vi "BT Rx Test Get Default LSL.vi"(8 "error in (no error)":errorcluster, 11 "Template Tx Test in":refnum<class "niDTS BT Rx Test.lvclass">) -> (0 "error out":errorcluster, 2 "Default LSL":T1, 3 "Template Tx Test out":refnum<class "niDTS BT Rx Test.lvclass">)   [LabVIEW 2015, in "niDTS BT.lvlib" / "niDTS BT Rx Test.lvclass"]
uses:
  niDTS BT Rx Test.lvclass
  Includes/niDTS BT Rx Test INC Results.ctl
  niDTS BT Rx Test.lvclass/niDTS BT Rx Test.ctl
  Includes/niDTS BT INC Standard.ctl
  Includes/niDTS BT Rx Test INC Default Limits.vi
  niDTS BT.lvlib
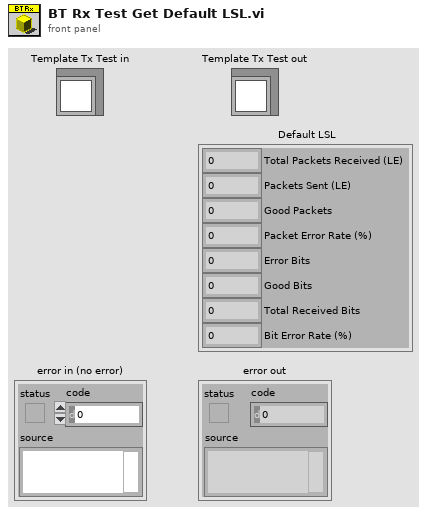
[diagram p1: front panel]
types:
  T1 = typedef "niDTS BT.lvlib/niDTS BT Rx Test INC Results.ctl" = cluster{"Total Packets Received (LE)":i32, "Packets Sent (LE)":dbl, "Good Packets":dbl, "Packet Error Rate (%)":dbl, "Error Bits":u32, "Good Bits":u32, "Total Received Bits":u32, "Bit Error Rate (%)":dbl}
  T2 = typedef "niDTS BT.lvlib/niDTS BT INC Standard.ctl" = enum16{"BDR", "EDR", "LE-TP"}
  T3 = typedef "niDTS BT.lvlib/niDTS BT INC Packet Type.ctl" = enum16{"NULL", "POLL", "FHS", "DM1", "DH1", "HV1", "HV2", "HV3", "EV3", "DV", "AUX1", "DM3", "DH3", "EV4", "EV5", "DM5", "DH5", "LE-TP"}
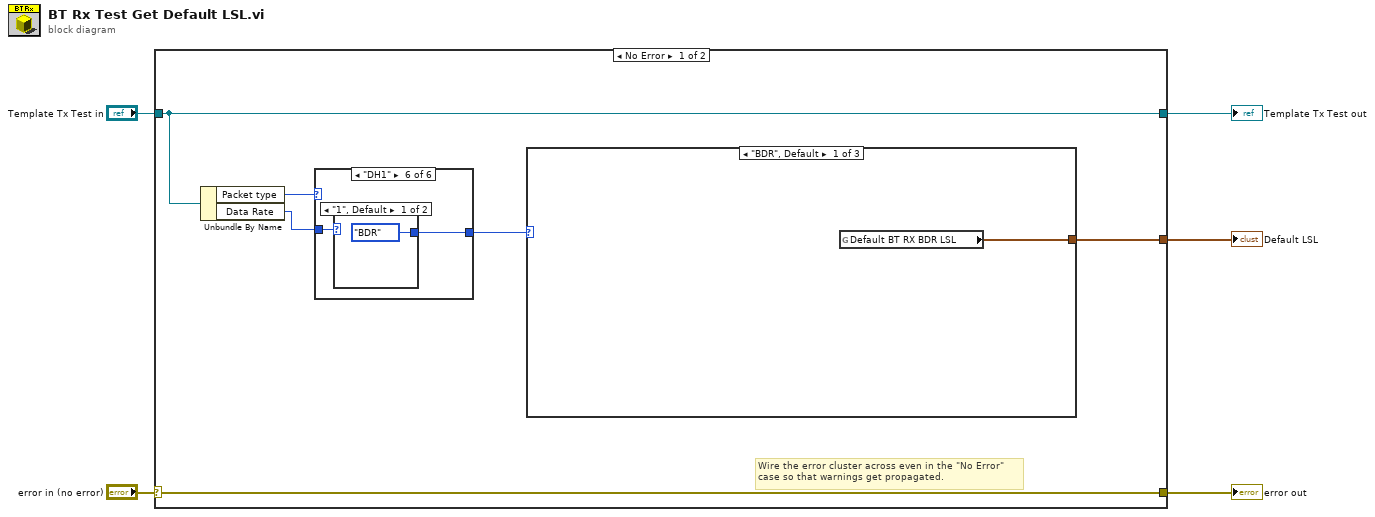
[diagram p0: block diagram]
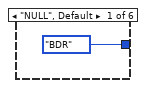
[diagram p2: hidden frame]
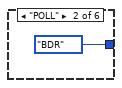
[diagram p3: hidden frame]
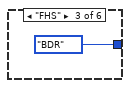
[diagram p4: hidden frame]
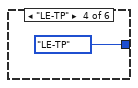
[diagram p5: hidden frame]
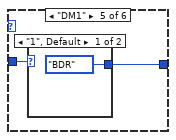
[diagram p6: hidden frame]
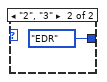
[diagram p7: hidden frame]
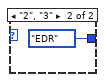
[diagram p8: hidden frame]
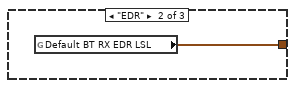
[diagram p9: hidden frame]
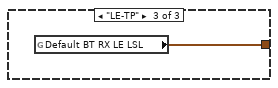
[diagram p10: hidden frame]
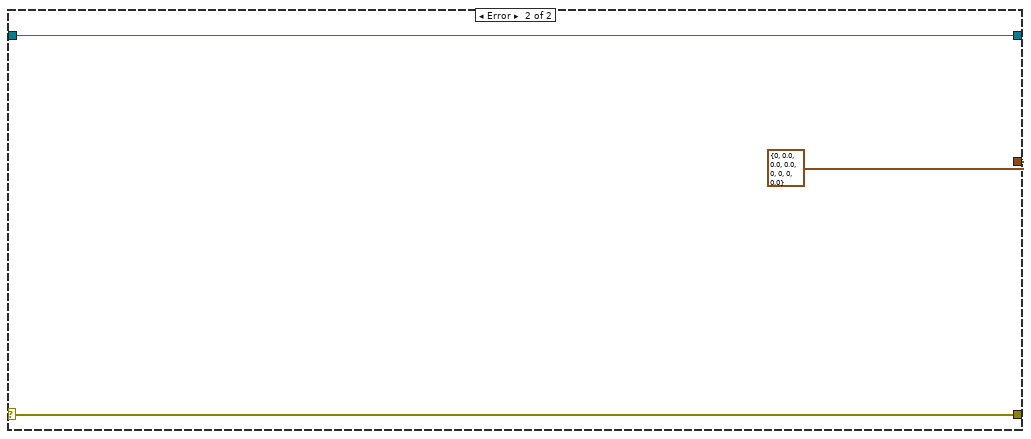
[diagram p11: hidden frame]
diagram:
  n1 = case shown="No Error" "error in (no error)" {
    selector: "error in (no error)" -> [w11 w29]
    tunnel: [w11 w29] -> w4
    tunnel: [w6 w28] -> w2
    tunnel: "Template Tx Test in" -> [w6 w28]
    tunnel: [w7 T1 {"Total Packets Received (LE)"=0, "Packets Sent (LE)"=0.0, "Good Packets"=0.0, "Packet Error Rate (%)"=0.0, "Error Bits"=0, "Good Bits"=0, "Total Received Bits"=0, "Bit Error Rate (%)"=0.0} ("Default LSL")] -> w1
    frame No Error {
      # "Wire the error cluster across even in the \"No Error\"\ncase so that warnings get propagated."
      n2 = Unbundle By Name(w6) -> ("Packet type"=w9:T3, "Data Rate"=w10:enum16{"1", "2", "3"})
      n3 = case shown="\"DH1\"" w9 {
        tunnel: w10 -> [_ _ _ _ w17 w21]
        tunnel: [niDTS_BT_INC_Standard."BDR" ("BT Standard") niDTS_BT_INC_Standard."BDR" ("BT Standard") niDTS_BT_INC_Standard."BDR" ("BT Standard") niDTS_BT_INC_Standard."LE-TP" ("BT Standard") w16 w20] -> w8
        frame "NULL", Default {
        }
        frame "POLL" {
        }
        frame "FHS" {
        }
        frame "LE-TP" {
        }
        frame "DM1" {
          n4 = case shown="\"1\", Default" w17 {
            tunnel: [niDTS_BT_INC_Standard."BDR" ("BT Standard") niDTS_BT_INC_Standard."EDR" ("BT Standard")] -> w16
            frame "1", Default {
            }
            frame "2", "3" {
            }
          }
        }
        frame "DH1" {
          n5 = case shown="\"1\", Default" w21 {
            tunnel: [niDTS_BT_INC_Standard."BDR" ("BT Standard") niDTS_BT_INC_Standard."EDR" ("BT Standard")] -> w20
            frame "1", Default {
            }
            frame "2", "3" {
            }
          }
        }
      }
      n6 = case shown="\"BDR\", Default" w8 {
        tunnel: [w24 w25 w26] -> w7
        frame "BDR", Default {
          n7 = global read "niDTS BT Rx Test INC Default Limits.vi" "Default BT RX BDR LSL"() -> (w24:T1)
        }
        frame "EDR" {
          n8 = global read "niDTS BT Rx Test INC Default Limits.vi" "Default BT RX EDR LSL"() -> (w25:T1)
        }
        frame "LE-TP" {
          n9 = global read "niDTS BT Rx Test INC Default Limits.vi" "Default BT RX LE LSL"() -> (w26:T1)
        }
      }
    }
    frame Error {
    }
  }
  "error out" <- w4
  "Template Tx Test out" <- w2
  "Default LSL" <- w1
